vi "Log Event.vi"(8 "error in (no error)":errorcluster, 10 "Event Text":string, 11 "SkynetCompiler in":refnum<class "LVAutomationListener.lvclass">) -> (0 "error out":errorcluster)   [LabVIEW 2013, in "LVAutomationListener.lvlib" / "LVAutomationListener.lvclass"]
doc: "Add text to the ongoing event log."
uses:
  LVAutomationListener.lvclass
  LVAutomationListener.lvclass/LVAutomationListener.ctl
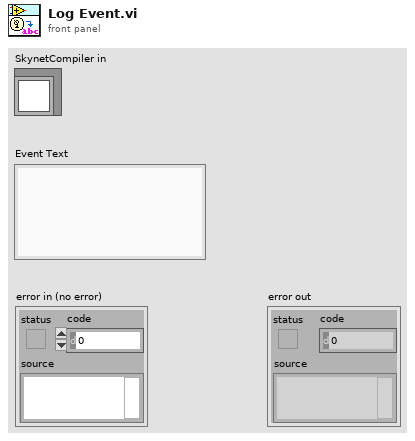
[diagram p1: front panel]
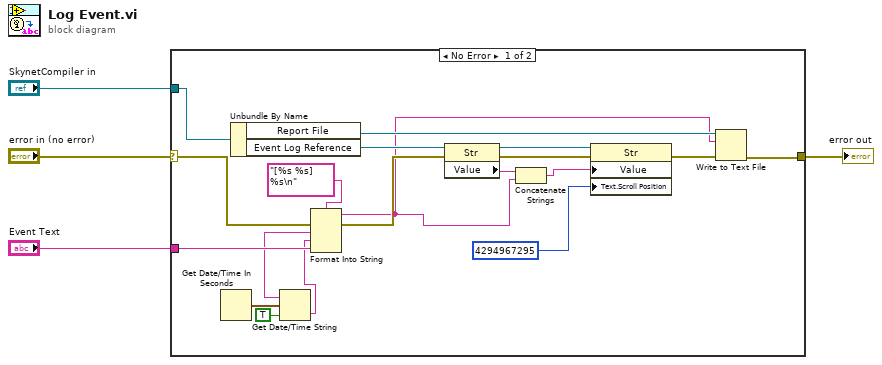
[diagram p0: block diagram]
diagram:
  n1 = case shown="No Error" "error in (no error)" {
    selector: "error in (no error)" -> [w12 w24]
    tunnel: [w14 w24] -> w3
    tunnel: "SkynetCompiler in" -> [w23 _]
    tunnel: "Event Text" -> [w9 _]
    frame No Error {
      n2 = Get Date/Time In Seconds() -> (seconds since 1Jan1904=w13:timestamp)
      n3 = Unbundle By Name(w23) -> ("Report File"=w15:refnum<file>, "Event Log Reference"=w22:refnum<vi>)
      n4 = Get Date/Time String(seconds (now)=w13, want seconds? (F)=TRUE) -> (date string=w8:string, time string=w7:string)  [unwired: 1 in]
      n5 = Format Into String(format string="[%s %s] %s\n" ("string"), error in=w12, w8, w7, w9) -> (resulting string=w6:string, error out=w11:errorcluster)  [unwired: 1 in]
      n6 = property class="Str"(reference=w22, error in=w11) -> (reference out=w21:refnum<vi>, error out=w20:errorcluster, "Value"=w17:string)
      n7 = Concatenate Strings(w17, w6) -> (w16:string)
      n8 = property class="Str"(reference=w21, error in=w20, "Value"=w16, "Text.Scroll Position"=u32 4294967295) -> (error out=w18:errorcluster)  [unwired: 1 out]
      n9 = Write to Text File(file (use dialog)=w15, text=w6, error in=w18) -> (error out=w14:errorcluster)  [unwired: 1 in, 2 out]
    }
    frame Error {
    }
  }
  "error out" <- w3
